vi "Read Configuration Parameters.vi"(8 "error in (no error)":errorcluster, 10 "refnum":T1, 11 "monitor configuration in":refnum<class "monitor configuration.lvclass">) -> (0 "error out":errorcluster, 2 "refnum out":T1, 3 "monitor configuration out":refnum<class "monitor configuration.lvclass">)   [LabVIEW 2016, in "Hardware.lvlib" / "monitor.lvlib" / "monitor configuration.lvclass"]
uses:
  <userlib>/Common Components/Hardware/Abstract System/Monitor/monitor configuration.lvclass
  <vilib>/Utility/config.llb/Config Data RefNum.ctl
  <userlib>/Configuration Dialog Actor/Configuration.lvclass
  <vilib>/Utility/config.llb/NI_LVConfig.lvlib
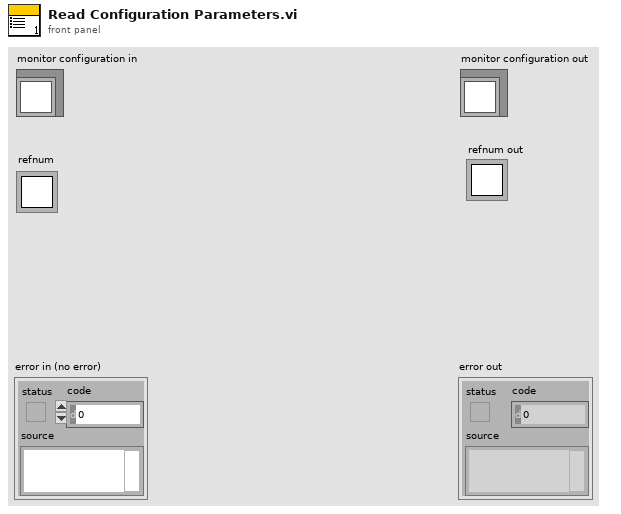
[diagram p1: front panel]
types:
  T1 = typedef "NI_LVConfig.lvlib/Config Data RefNum.ctl" = refnum<k1>
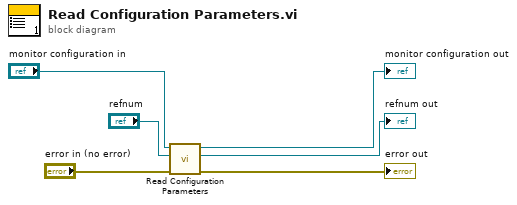
[diagram p0: block diagram]
diagram:
  n1 = call-parent "Read Configuration Parameters.vi"("error in (no error)"="error in (no error)", "refnum"="refnum", "Configuration in"="monitor configuration in") -> ("error out"=→"error out":errorcluster, "refnum out"=→"refnum out":T1, "Configuration out"=→"monitor configuration out":refnum<class "monitor configuration.lvclass">)  [unwired: 6 in]
